vi "COMMUNICATION_SETTING.vi"(7 "communication path":path, 8 "error in":errorcluster, 11 "STATION":string) -> (0 "error out":errorcluster, 2 "SCAN_COM":string, 3 "PRINT_COM":string)   [LabVIEW 2017]
uses:
  <vilib>/Utility/config.llb/Read Key (String).vi
  <vilib>/Utility/config.llb/NI_LVConfig.lvlib
panel:
  # "COMMUNICATION SETTING"
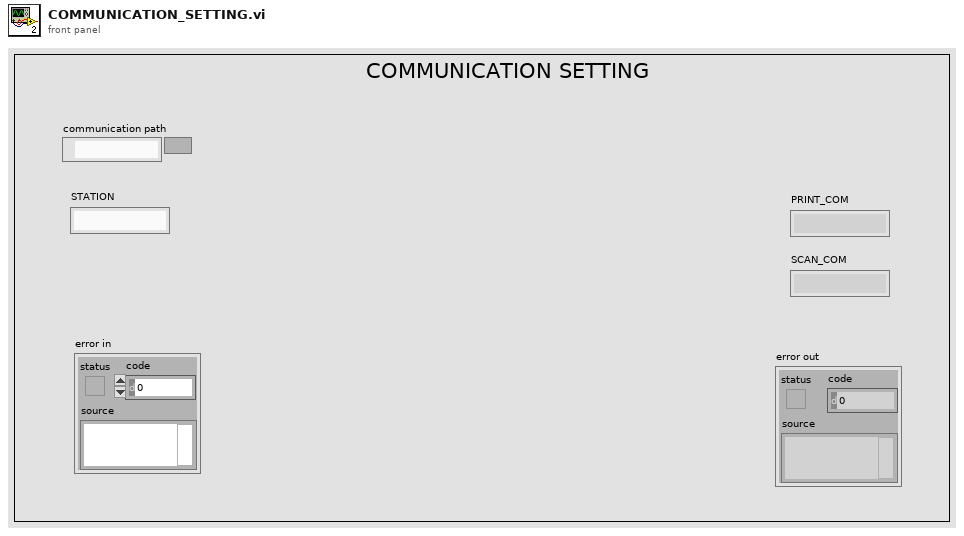
[diagram p1: front panel]
types:
  T1 = typedef "NI_LVConfig.lvlib/Config Data RefNum.ctl" = refnum<k1>
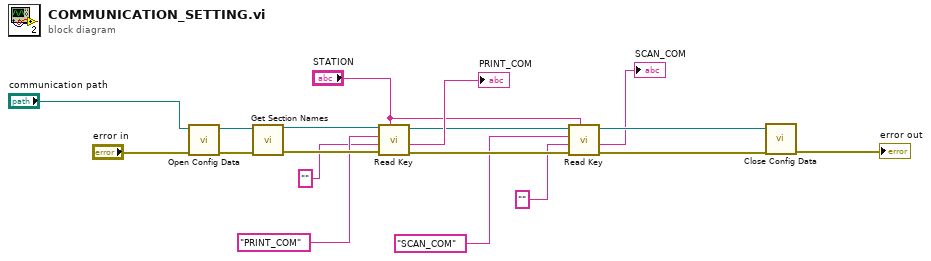
[diagram p0: block diagram]
diagram:
  n1 = call <vilib>:"Open Config Data.vi"("error in (no error)"="error in", "configuration file path"="communication path") -> ("error out"=w17:errorcluster, "refnum"=w18:T1)  [unwired: 7 in, 1 out]
  n2 = call <vilib>:"Get Section Names.vi"("error in (no error)"=w17, "refnum"=w18) -> ("error out"=w14:errorcluster, "refnum out"=w13:T1)  [unwired: 7 in, 1 out]
  n3 = call-poly <vilib>:"Read Key.vi"("section"="STATION", "error in (no error)"=w14, "default value"="", "key"="PRINT_COM" ("COM"), "refnum"=w13) -> ("error out"=w10:errorcluster, "value"=→"PRINT_COM":string, "refnum out"=w8:T1)  [unwired: 3 in, 1 out]
  n4 = call-poly <vilib>:"Read Key.vi"("section"="STATION", "error in (no error)"=w10, "default value"="", "key"="SCAN_COM" ("COM"), "refnum"=w8) -> ("error out"=w9:errorcluster, "value"=→"SCAN_COM":string, "refnum out"=w7:T1)  [unwired: 3 in, 1 out]
  n5 = call <vilib>:"Close Config Data.vi"("error in (no error)"=w9, "refnum"=w7) -> ("error out"=→"error out":errorcluster)  [unwired: 8 in, 1 out]
